vi "timestamp to datestamp.vi"(8 "error in":errorcluster, 11 "time stamp":timestamp) -> (0 "error out":errorcluster, 3 "remaining string":string)   [LabVIEW 2014]
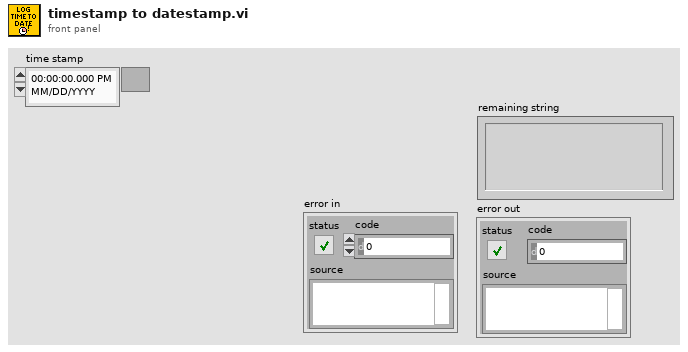
[diagram p1: front panel]
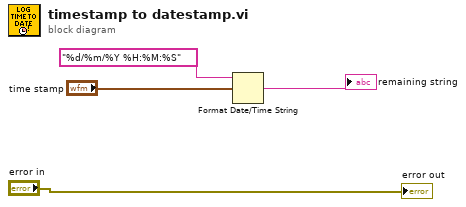
[diagram p0: block diagram]
diagram:
  n1 = Format Date/Time String(time format string (%c)="%d/%m/%Y %H:%M:%S", seconds (now)="time stamp") -> (date/time string=→"remaining string":string)  [unwired: 1 in]
  "error out" <- "error in"
